vi "executeDuelistSkill.vi"(8 "error in (no error)":errorcluster, 9 "Duelist Robot in":refnum<class "Robot.lvclass">, 10 "Game":refnum<class "Game.lvclass">, 11 "DuelistSkill in":refnum<class "DuelistSkill.lvclass">) -> (0 "error out":errorcluster, 1 "Duelist Robot out":refnum<class "Robot.lvclass">, 3 "DuelistSkill out":refnum<class "DuelistSkill.lvclass">)   [LabVIEW 2023, in "DuelistSkill.lvclass"]
uses:
  DuelistSkill.lvclass
  Game_class/Game.lvclass
  Robot_class/Robot.lvclass
  C:/Users/ebert/Desktop/roboime/SSL_AI/Object_class/Object.lvclass
  Utilities_class/Utilities.lvclass
  Game_class/Game.lvclass/Game.ctl
  Team_class/Team.lvclass/Team.ctl
  Object_class/Object.lvclass/Object.ctl
  Game_class/Read FieldRef.vi
  Game_class/Read EnemyRef.vi
  Game_class/Read DefensiveTeam.vi
  Game_class/Read BallRef.vi
  Team_class/Read RobotRef.vi
  Object_class/Read x.vi
  Object_class/Read y.vi
  Enemy_class/Enemy.lvclass
  C:/Users/ebert/Desktop/roboime/SSL_AI/Team_class/Team.lvclass
  Ally_class/Ally.lvclass
  Ball_class/Ball.lvclass
  Field_class/Field.lvclass
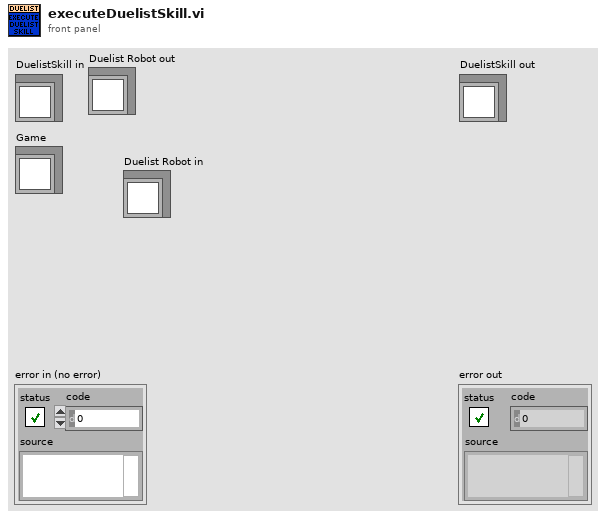
[diagram p1: front panel]
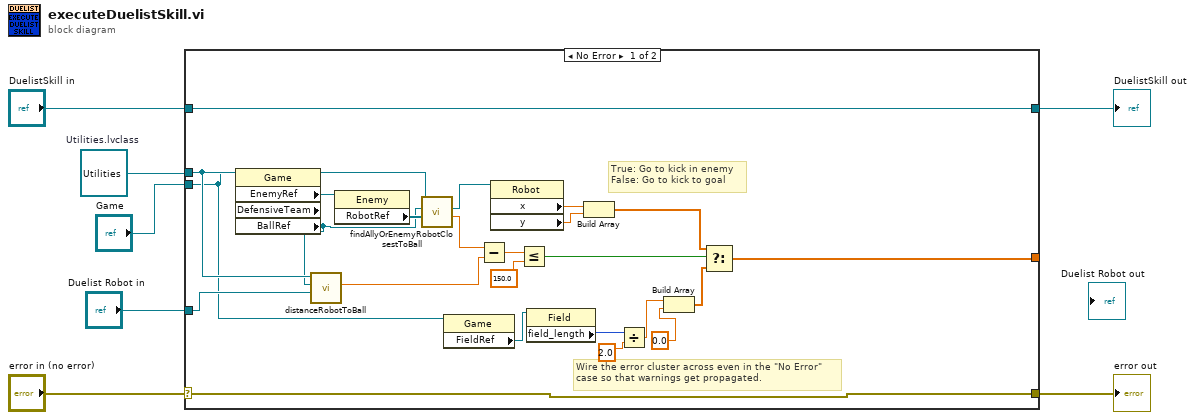
[diagram p0: block diagram]
diagram:
  w3 = refnum<class "Utilities.lvclass"> refnum  # Utilities.lvclass
  n1 = case shown="No Error" "error in (no error)" {
    selector: "error in (no error)" -> [w30 w33]
    tunnel: [w30 w33] -> w6
    tunnel: [w31 w32] -> w4
    tunnel: "DuelistSkill in" -> [w31 w32]
    tunnel: w3 -> [w27 _]
    tunnel: "Game" -> [w16 _]
    tunnel: "Duelist Robot in" -> [w26 _]
    tunnel: [w9 _] -> _
    frame No Error {
      # "True: Go to kick in enemy\nFalse: Go to kick to goal"
      # "Wire the error cluster across even in the \"No Error\"\ncase so that warnings get propagated."
      n2 = property class="Game" props=["EnemyRef", "DefensiveTeam", "BallRef"](reference=w16) -> ("EnemyRef"=w29:refnum<class "Enemy.lvclass">, "BallRef"=w8:refnum<class "Ball.lvclass">)  [unwired: 1 in, 3 out]
      n3 = call "distanceRobotToBall.vi"("Robot"=w26, "Ball"=w8, "Utilities in"=w27) -> ("Distance Robot To Ball"=w24:dbl)  [unwired: 6 in, 2 out]
      n4 = property class="Enemy"(reference=w29) -> ("RobotRef"=w28:refnum<class "Robot.lvclass">[])  [unwired: 1 in, 2 out]
      n5 = call "findAllyOrEnemyRobotClosestToBall.vi"("Ally/Enemy Robots"=w28, "Ball"=w8, "Utilities in"=w27) -> ("Robot distance to ball"=w25:dbl, "Robot"=w20:refnum<class "Robot.lvclass">)  [unwired: 4 in, 3 out]
      n6 = property class="Game"(reference=w16) -> ("FieldRef"=w15:refnum<class "Field.lvclass">)  [unwired: 1 in, 2 out]
      n7 = Subtract(x=w25, y=w24) -> (x-y=w23:dbl)
      n8 = property class="Robot"(reference=w20) -> ("x"=w19:dbl, "y"=w18:dbl)  [unwired: 1 in, 2 out]
      n9 = Less Or Equal?(x=w23, y=150.0) -> (x <= y?=w21:bool)
      n10 = property class="Field"(reference=w15) -> ("field_length"=w14:i32)  [unwired: 1 in, 2 out]
      n11 = Build Array(w19, w18) -> (w17:dbl[])
      n12 = Divide(x=w14, y=2.0 ("field_length")) -> (x/y=w12:dbl)
      n13 = Build Array(w12, 0.0 ("field_length")) -> (w10:dbl[])
      n14 = Select(t=w17, s=w21, f=w10) -> (s? t:f=w9:dbl[])
    }
    frame Error {
    }
  }
  "error out" <- w6
  "DuelistSkill out" <- w4
